vi "X_normalized.vi"(1 "X":T1) -> (0 "X_normalized":T1)   [LabVIEW 2016]
uses:
  <vilib>/Analysis/Matrix/Datatypes/RealMatrix.ctl
  <vilib>/Analysis/Matrix/Numeric/Conversions/Matrix To Array - RM.vi
  <vilib>/Analysis/Matrix/Numeric/Conversions/Array To Matrix - RA2.vi
  <vilib>/Analysis/Matrix/NI_Matrix.lvlib
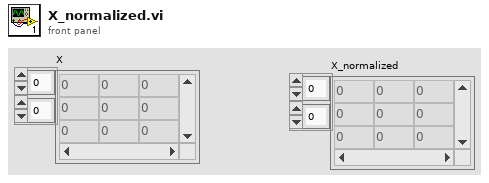
[diagram p1: front panel]
types:
  T1 = typedef "NI_Matrix.lvlib/RealMatrix.ctl" = dbl[][]
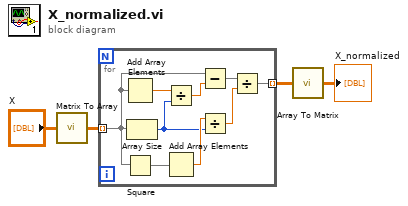
[diagram p0: block diagram]
diagram:
  n1 = call-poly <vilib>:"Matrix To Array.vi"("Real Matrix"="X") -> ("Real 2D Array"=w3:dbl[][])
  n2 = for {
    tunnel: w3 -> [w11] mode=indexing
    tunnel: [w5] -> w2 mode=indexing
    n3 = Add Array Elements(numeric array=w11) -> (sum=w13:dbl)
    n4 = Square(x=w11) -> (x^2=w10:dbl[])
    n5 = Array Size(array=w11) -> (size(s)=w8:i32)
    n6 = Divide(x=w13, y=w8) -> (x/y=w12:dbl)
    n7 = Add Array Elements(numeric array=w10) -> (sum=w9:dbl)
    n8 = Subtract(x=w11, y=w12) -> (x-y=w7:dbl[])
    n9 = Divide(x=w9, y=w8) -> (x/y=w6:dbl)
    n10 = Divide(x=w7, y=w6) -> (x/y=w5:dbl[])
  }
  n11 = call-poly <vilib>:"Array To Matrix.vi"("Real 2D Array"=w2) -> ("Real Matrix"=→"X_normalized":T1)
